vi "Clear.vi"(8 "error in (no error)":errorcluster, 11 "ResultTree in":refnum<class "Result Tree.lvclass">) -> (0 "error out":errorcluster, 3 "ResultTree out":refnum<class "Result Tree.lvclass">)   [LabVIEW 2017, in "Result Tree.lvclass"]
doc: "Removes all items from the tree."
uses:
  Result Tree.lvclass
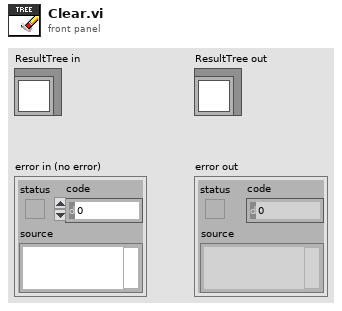
[diagram p1: front panel]
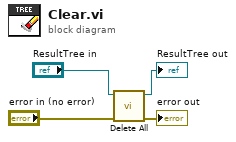
[diagram p0: block diagram]
diagram:
  n1 = call "Delete All.vi"("error in (no error)"="error in (no error)", "ResultTree in"="ResultTree in") -> ("error out"=→"error out":errorcluster, "ResultTree out"=→"ResultTree out":refnum<class "Result Tree.lvclass">)  [unwired: 8 in]
